vi "MTM2_getEvent_largeFileObjectAvailable.vi"(8 "error in (no error)":errorcluster, 11 "logevent_largeFileObjectAvailable_Ctl":T1={"private_rcvStamp"=0.0, "url"="                                                                                                                                                                                                                                                                ", "generator"="", "version"=0.0, "byteSize"=0, "checkSum"="                                                                                                                                                                                                                                                                ", "mimeType"="                                                                                                                                                                                                                                                                ", "id"="                                                                                                                                                                                                                                                                ", "priority"=0}) -> (0 "error out":errorcluster, 2 "function return":i32, 3 "logevent_largeFileObjectAvailable_Ctl out":T1={"private_rcvStamp"=0.0, "url"="                                                                                                                                                                                                                                                                ", "generator"="", "version"=0.0, "byteSize"=0, "checkSum"="                                                                                                                                                                                                                                                                ", "mimeType"="                                                                                                                                                                                                                                                                ", "id"="                                                                                                                                                                                                                                                                ", "priority"=0})   [LabVIEW 2018, in "SALLV_MTM2.lvlib"]
doc: "int MTM2_shm_getEvent_largeFileObjectAvailableLV(MTM2_logevent_largeFileObjectAvailableLV *logevent_largeFileObjectAvailable_Ctl );"
uses:
  DataTypes/logevent_largeFileObjectAvailable.ctl
  SALLV_MTM2.lvlib
  SALLV_MTM2.so
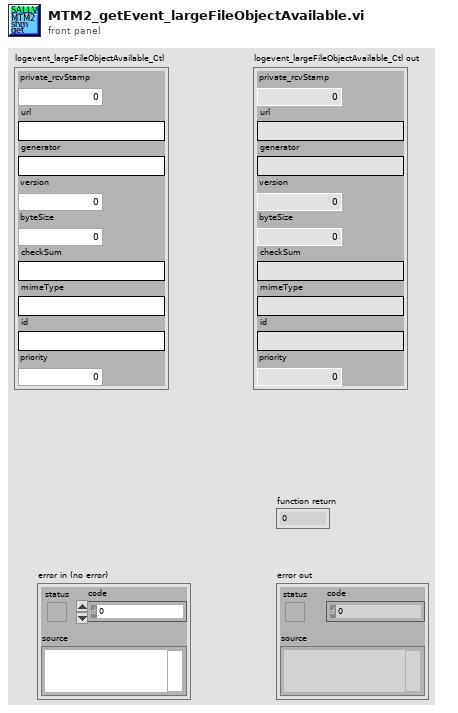
[diagram p1: front panel]
types:
  T1 = typedef "SALLV_MTM2.lvlib/logevent_largeFileObjectAvailable.ctl" = cluster{"private_rcvStamp":dbl, "url":string, "generator":string, "version":sgl, "byteSize":i32, "checkSum":string, "mimeType":string, "id":string, "priority":i32}
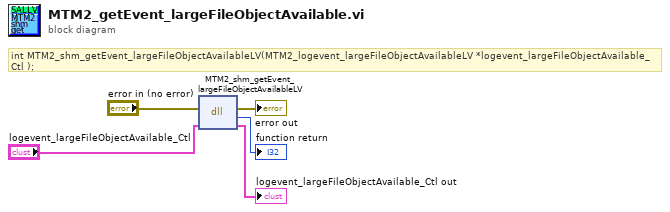
[diagram p0: block diagram]
diagram:
  # "int MTM2_shm_getEvent_largeFileObjectAvailableLV(MTM2_logevent_largeFileObjectAvailableLV *logevent_largeFileObjectAvailable_Ctl );"
  n1 = dll-call lib="home/ttsai/Documents/salLabviewApi/SALLV_MTM2/SALLV_MTM2.*" fn="MTM2_shm_getEvent_largeFileObjectAvailableLV"(error in="error in (no error)", "logevent_largeFileObjectAvailable_Ctl"="logevent_largeFileObjectAvailable_Ctl") -> (error out=→"error out":errorcluster, →"function return":i32, "logevent_largeFileObjectAvailable_Ctl"=→"logevent_largeFileObjectAvailable_Ctl out":T1)  [unwired: 2 in, 1 out]
